vi "Verify Row  for Standard Table[  ].vi"(0 "Table size":cluster{"# Column":u16, "# Row":u16}, 7 "Borders IN":T1) -> (8 "Borders OUT":T1)   [LabVIEW 2019]
doc: "Developed by Jean-Marc Simard\nCopyright © 2012, Exaprom Inc.\nAll rights reserved.\nLicense: BSD\n\nWith iTextSharp 4.1.6 (http://itextsharp.sourceforge.net)\nunder Mozilla Public License Version 1.1\n(http://www.mozilla.org/MPL/MPL-1.1.html)"
uses:
  <userlib>/Exaprom PDF/Controls/Table Controls/Simplified Table Row Borders [ ].ctl
  <userlib>/Exaprom PDF/Controls/Table Controls/Simplified Table Row Borders.ctl
  <userlib>/Exaprom PDF/Controls/Table Controls/Border and BG Color [ ].ctl
  <userlib>/Exaprom PDF/Controls/Table Controls/Border and BG Color.ctl
  <userlib>/Exaprom PDF/Controls/Table Controls/Cell Border 20 px.ctl
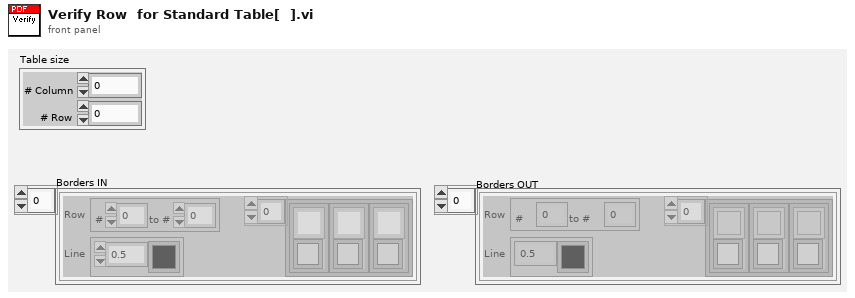
[diagram p1: front panel]
types:
  T1 = typedef "Simplified Table Row Borders [ ].ctl" = T2[]
  T2 = typedef "Simplified Table Row Borders.ctl" = cluster{"Row":cluster{"#":i16, "to #":i16}, "Line":cluster{"Thickness":sgl, "Color":u32}, "Column Borders [ ]":T3}
  T3 = typedef "Border and BG Color [ ].ctl" = T4[]
  T4 = typedef "Border and BG Color.ctl" = cluster{"Cell Border":T5, "BG":u32}
  T5 = typedef "Cell Border 20 px.ctl" = u16
  T6 = cluster{cluster{"Row.to #":i16, u16}, "Line":cluster{"Thickness":sgl, "Color":u32}, "Column Borders [ ]":T3}
  T7 = cluster{cluster{"#":i16, "to #":i16}, "Line":cluster{"Thickness":sgl, "Color":u32}, "Column Borders [ ]":T3}
  T8 = cluster{cluster{"#":u16, "#":u16}, "Line":cluster{"Thickness":sgl, "Color":u32}, "Column Borders [ ]":T3}
  T9 = cluster{"Row":cluster{"#":i16, "to #":i16}, "Line":cluster{"Thickness":sgl, "Color":u32}, "Column Borders [ ]":T3}
  T10 = cluster{"Row":cluster{"#":i16, "to #":i16}, "Line":cluster{"Thickness":sgl, "Color":u32}, T3}
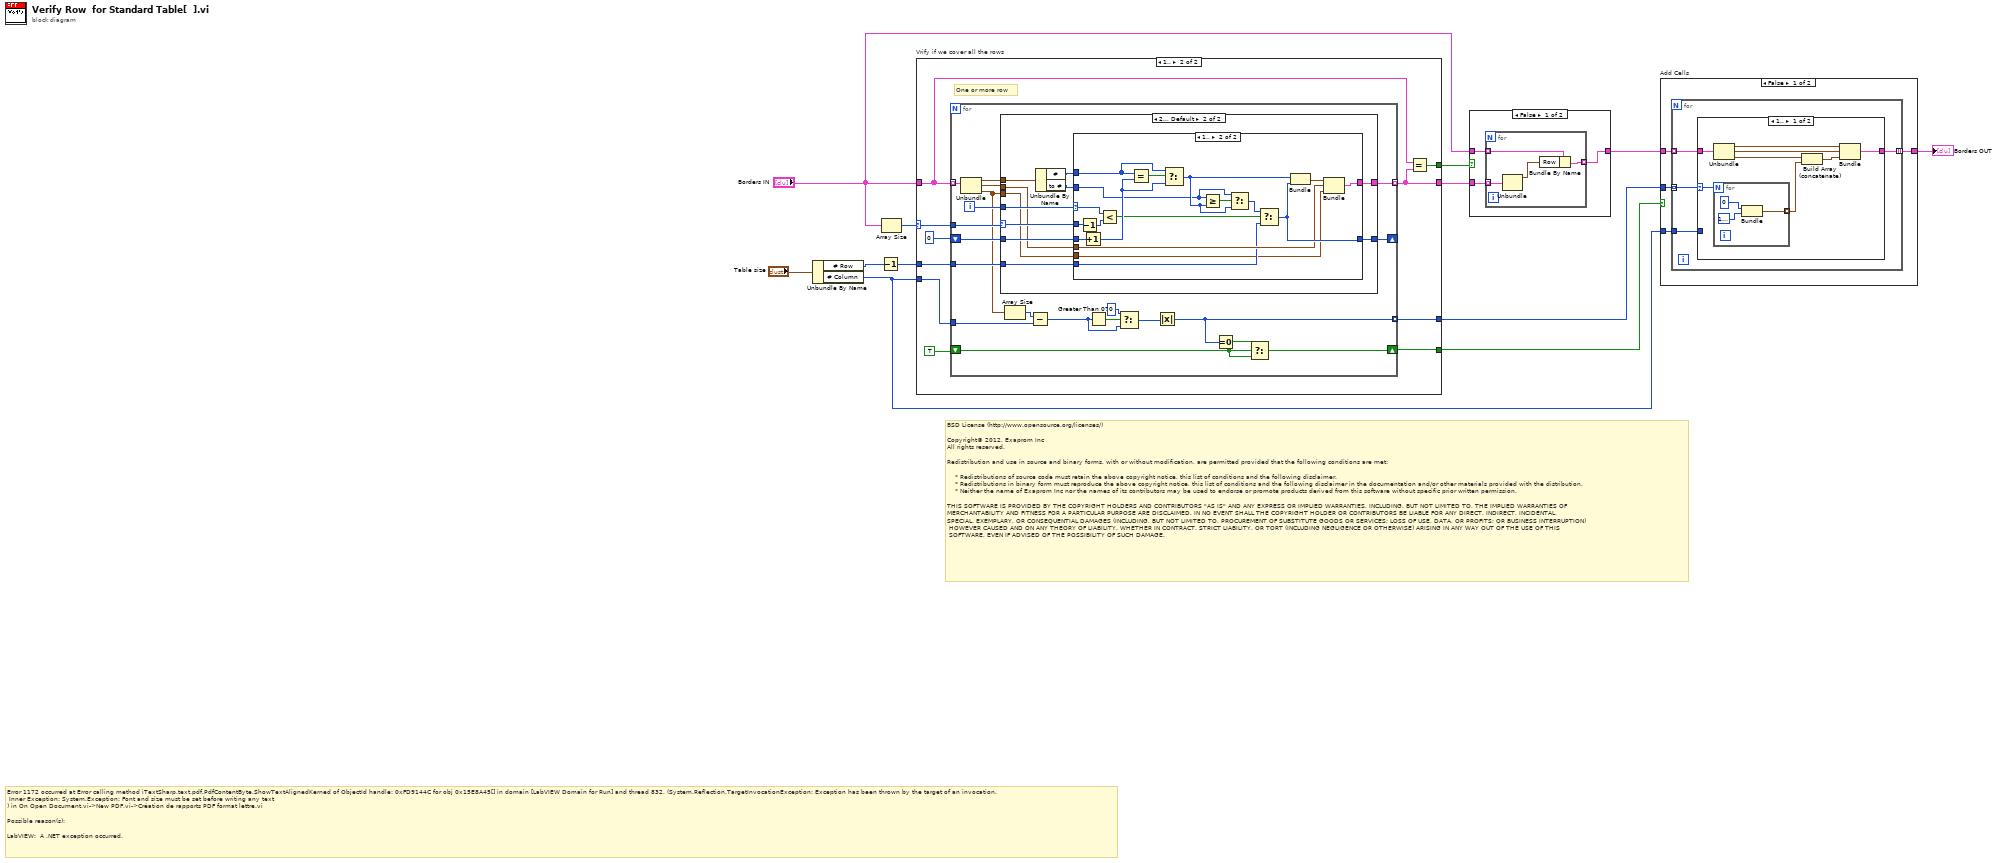
[diagram p0: block diagram]
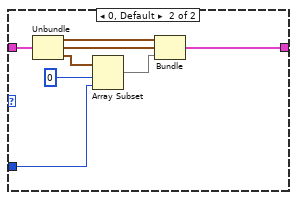
[diagram p2: hidden frame]
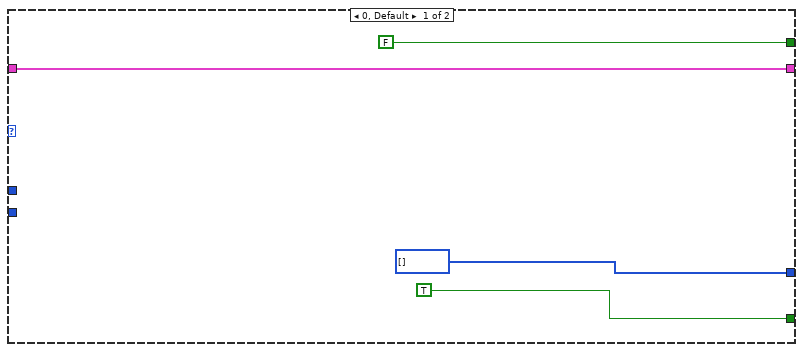
[diagram p5: hidden frame]
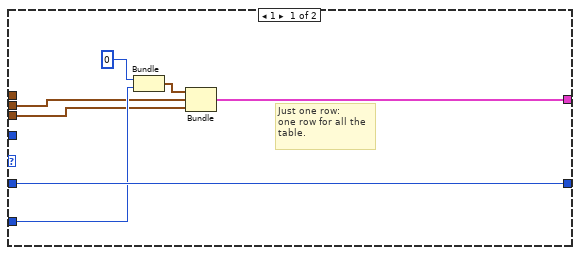
[diagram p6: hidden frame]
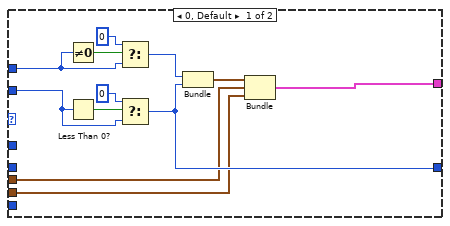
[diagram p7: hidden frame]
diagram:
  # "Error 1172 occurred at Error calling method iTextSharp.text.pdf.PdfContentByte.ShowTextAlignedKerned of ObjectId handle: 0xFD9144C for obj 0x15E8A45[] in domain [LabVIEW Domain for Run] and thread 832, (System.Reflection.TargetInvocationException: Exception has been thrown by the target of an invocation.\n\tInner Exception: System.Exception: Font and size must be set before writing any text\n) in On Open Document.vi->New PDF.vi->Création de rapports PDF format lettre.vi\n\nPossible reason(s):\n\nLabVIEW:  A .NET exception occurred."
  # "BSD License (http://www.opensource.org/licenses/)\n\nCopyright© 2012, Exaprom Inc\nAll rights reserved.\n\nRedistribution and use in source and binary forms, with or without modification, are permitted provided that the following conditions are met:\n\n    * Redistributions of source code must retain the above copyright notice, this list of conditions and the following disclaimer.\n    * Redistributions in binary form must reproduce the above copyright notice, this list of conditions and the following disclaimer in the documentation and/or other materials provided with the distribution.\n    * Neither the name of Exaprom Inc nor the names of its contributors may be used to endorse or promote products derived from this software without specific prior written permission.\n\nTHIS SOFTWARE IS PROVIDED BY THE COPYRIGHT HOLDERS AND CONTRIBUTORS \"AS IS\" AND ANY EXPRESS OR IMPLIED WARRANTIES, INCLUDING, BUT NOT LIMITED TO, THE IMPLIED WARRANTIES OF \nMERCHANTABILITY AND FITNESS FOR A PARTICULAR PURPOSE ARE DISCLAIMED. IN NO EVENT SHALL THE COPYRIGHT HOLDER OR CONTRIBUTORS BE LIABLE FOR ANY DIRECT, INDIRECT, INCIDENTAL,\nSPECIAL, EXEMPLARY, OR CONSEQUENTIAL DAMAGES (INCLUDING, BUT NOT LIMITED TO, PROCUREMENT OF SUBSTITUTE GOODS OR SERVICES; LOSS OF USE, DATA, OR PROFITS; OR BUSINESS INTERRUPTION)\n HOWEVER CAUSED AND ON ANY THEORY OF LIABILITY, WHETHER IN CONTRACT, STRICT LIABILITY, OR TORT (INCLUDING NEGLIGENCE OR OTHERWISE) ARISING IN ANY WAY OUT OF THE USE OF THIS\n SOFTWARE, EVEN IF ADVISED OF THE POSSIBILITY OF SUCH DAMAGE."
  n1 = Unbundle By Name("Table size") -> ("# Row"=w8:u16, "# Column"=w1:u16)
  n2 = Decrement(x=w8) -> (x-1=w7:u16)
  n3 = Array Size(array="Borders IN") -> (size(s)=w12:i32)
  n4 = case "Vrify if we cover all the rows" shown="1.." w12 {
    selector: w12 -> [_ w26]
    tunnel: "Borders IN" -> [w15 w23]
    tunnel: [w15 w24] -> w10
    tunnel: [FALSE w22] -> w11
    tunnel: w7 -> [_ w21]
    tunnel: w1 -> [_ w20]
    tunnel: [i32[] [] w19] -> w5
    tunnel: [TRUE w17] -> w3
    frame 0, Default {
    }
    frame 1.. {
      # "One or more row"
      n5 = for {
        tunnel: w23 -> [w42] mode=indexing
        tunnel: w26 -> [w46]
        shift-right: [w44] -> _
        shift-left: i16 0 ("t") -> [w43]
        tunnel: [w40] -> w24 mode=indexing
        tunnel: w21 -> [w39]
        tunnel: w20 -> [w35]
        tunnel: [w31] -> w19 mode=indexing
        shift-right: [w34] -> w17
        shift-left: TRUE -> [w33]
        i -> [w45]
        n6 = Unbundle(w42) -> ("Row"=w41:cluster{"#":i16, "to #":i16}, "Line"=w38:cluster{"Thickness":sgl, "Color":u32}, "Column Borders [ ]"=w37:T3)
        n7 = case shown="2.., Default" w46 {
          selector: w46 -> [_ w60]
          tunnel: w45 -> [_ w64]
          tunnel: [w50 w63] -> w40
          tunnel: [w52 w62] -> w44
          tunnel: w43 -> [w52 w61]
          tunnel: w41 -> [_ w57]
          tunnel: w39 -> [w49 w56]
          tunnel: w38 -> [w48 w55]
          tunnel: w37 -> [w47 w54]
          frame 1 {
            # "Just one row: \none row for all the\ntable."
            n8 = Bundle("Row.to #"=i16 0, w49) -> (w51:cluster{"Row.to #":i16, u16})  [unwired: 1 in]
            n9 = Bundle(w51, "Line"=w48, "Column Borders [ ]"=w47) -> (w50:T6)  [unwired: 1 in]
          }
          frame 2.., Default {
            n10 = Unbundle By Name(w57) -> ("#"=w59:i16, "to #"=w58:i16)
            n11 = case shown="1.." w64 {
              selector: w64 -> [_ w86]
              tunnel: w59 -> [w75 w91]
              tunnel: w58 -> [w71 w88]
              tunnel: [w68 w80] -> w63
              tunnel: [w69 w82] -> w62
              tunnel: w61 -> [_ w92]
              tunnel: w60 -> [_ w87]
              tunnel: w55 -> [w66 w79]
              tunnel: w56 -> [_ w78]
              tunnel: w54 -> [w65 w77]
              frame 0, Default {
                n12 = Not Equal To 0?(x=w75) -> (x != 0?=w76:bool)
                n13 = Less Than 0?(x=w71) -> (x < 0?=w72:bool)
                n14 = Select(t=i16 0, s=w76, f=w75) -> (s? t:f=w70:i16)
                n15 = Select(t=i16 0, s=w72, f=w71) -> (s? t:f=w69:i16)
                n16 = Bundle("#"=w70, "to #"=w69) -> (w67:cluster{"#":i16, "to #":i16})  [unwired: 1 in]
                n17 = Bundle(w67, "Line"=w66, "Column Borders [ ]"=w65) -> (w68:T7)  [unwired: 1 in]
              }
              frame 1.. {
                n18 = Decrement(x=w87) -> (x-1=w85:i32)
                n19 = Increment(x=w92) -> (x+1=w90:u16)
                n20 = Less?(x=w86, y=w85) -> (x < y?=w83:bool)
                n21 = Equal?(x=w91, y=w90) -> (x = y?=w94:bool)
                n22 = Select(t=w91, s=w94, f=w90) -> (s? t:f=w89:u16)
                n23 = Greater Or Equal?(x=w88, y=w89) -> (x >= y?=w93:bool)
                n24 = Select(t=w88, s=w93, f=w89) -> (s? t:f=w84:u16)
                n25 = Select(t=w84, s=w83, f=w78) -> (s? t:f=w82:u16)
                n26 = Bundle("#"=w89, "#"=w82) -> (w81:cluster{"#":u16, "#":u16})  [unwired: 1 in]
                n27 = Bundle(w81, "Line"=w79, "Column Borders [ ]"=w77) -> (w80:T8)  [unwired: 1 in]
              }
            }
          }
        }
        n28 = Array Size(array=w37) -> (size(s)=w36:i32)
        n29 = Subtract(x=w36, y=w35) -> (x-y=w29:i32)
        n30 = Greater Than 0?(x=w29) -> (x > 0?=w30:bool)
        n31 = Select(t=0, s=w30, f=w29) -> (s? t:f=w27:i32)
        n32 = Absolute Value(x=w27) -> (abs(x)=w31:i32)
        n33 = Equal To 0?(x=w31) -> (x = 0?=w32:bool)
        n34 = Select(t=w32, s=w33, f=w33) -> (s? t:f=w34:bool)
      }
      n35 = Equal?(x=w23, y=w24) -> (x = y?=w22:bool)
    }
  }
  n36 = case shown="False" w11 {
    tunnel: w10 -> [w96 _]
    tunnel: "Borders IN" -> [w97 w102]
    tunnel: [w95 w102] -> w4
    frame False {
      n37 = for {
        tunnel: w97 -> [w101] mode=indexing
        tunnel: w96 -> [w100] mode=indexing
        tunnel: [w98] -> w95 mode=indexing
        n38 = Unbundle(w100) -> ("Row"=w99:cluster{"#":u16, "#":u16})  [unwired: 2 out]
        n39 = Bundle By Name(cluster=w101, "Row"=w99) -> (w98:T2)
      }
    }
    frame True {
    }
  }
  n40 = case "Add Cells" shown="False" w3 {
    tunnel: w5 -> [w106 _]
    tunnel: w4 -> [w105 w130]
    tunnel: [w104 w130] -> w2
    tunnel: w1 -> [w103 _]
    frame False {
      n41 = for {
        tunnel: w106 -> [w109] mode=indexing
        tunnel: w105 -> [w110] mode=indexing
        tunnel: [w108] -> w104 mode=indexing
        tunnel: w103 -> [w107]
        n42 = case shown="1.." w109 {
          selector: w109 -> [w117 _]
          tunnel: w110 -> [w118 w129]
          tunnel: [w116 w128] -> w108
          tunnel: w107 -> [_ w122]
          frame 1.. {
            n43 = Unbundle(w118) -> ("Row"=w114:cluster{"#":i16, "to #":i16}, "Line"=w115:cluster{"Thickness":sgl, "Color":u32}, "Column Borders [ ]"=w113:T3)
            n44 = for {
              N: w117 -> [_]
              tunnel: [w119] -> w112 mode=indexing
              n45 = Bundle("Cell Border 2"=T5 0, "BG"=u32 16777225) -> (w119:cluster{"Cell Border 2":T5, "BG":u32})  [unwired: 1 in]
            }
            n46 = Build Array (concatenate)(w113, w112) -> (w111:T3)
            n47 = Bundle("Row"=w114, "Line"=w115, "Column Borders [ ]"=w111) -> (w116:T9)  [unwired: 1 in]
          }
          frame 0, Default {
            n48 = Unbundle(w129) -> ("Row"=w126:cluster{"#":i16, "to #":i16}, "Line"=w127:cluster{"Thickness":sgl, "Color":u32}, "Column Borders [ ]"=w125:T3)
            n49 = Array Subset(array=w125, index=0, length=w122) -> (w124:T3)
            n50 = Bundle("Row"=w126, "Line"=w127, w124) -> (w128:T10)  [unwired: 1 in]
          }
        }
      }
    }
    frame True {
    }
  }
  "Borders OUT" <- w2
